vi "roboLV.vi"() -> ()   [LabVIEW 2013]
uses:
  <vilib>/Instr/_visa.llb/VISA Configure Serial Port (Instr).vi
panel:
  out "Elbow Waveform":dbl(graph)
  out "Elbow":dbl[](array[numeric])
  out "Gripper":bool
  out "Wrist":bool
  out "Elbow":bool
  out "Shoulder":bool
  out "Base":bool
  out "Wrist Waveform":dbl(graph)
  out "Shoulder Waveform":dbl(graph)
  out "String":string
  out "Numeric":dbl
  out "Wrist":dbl[](array[numeric])
  out "Shoulder":dbl[](array[numeric])
  in  "Clear":bool
  in  "?":bool
  out "?":bool
  out "Motor":u32
  in  "VISA resource name":refnum<visa-resource-name>
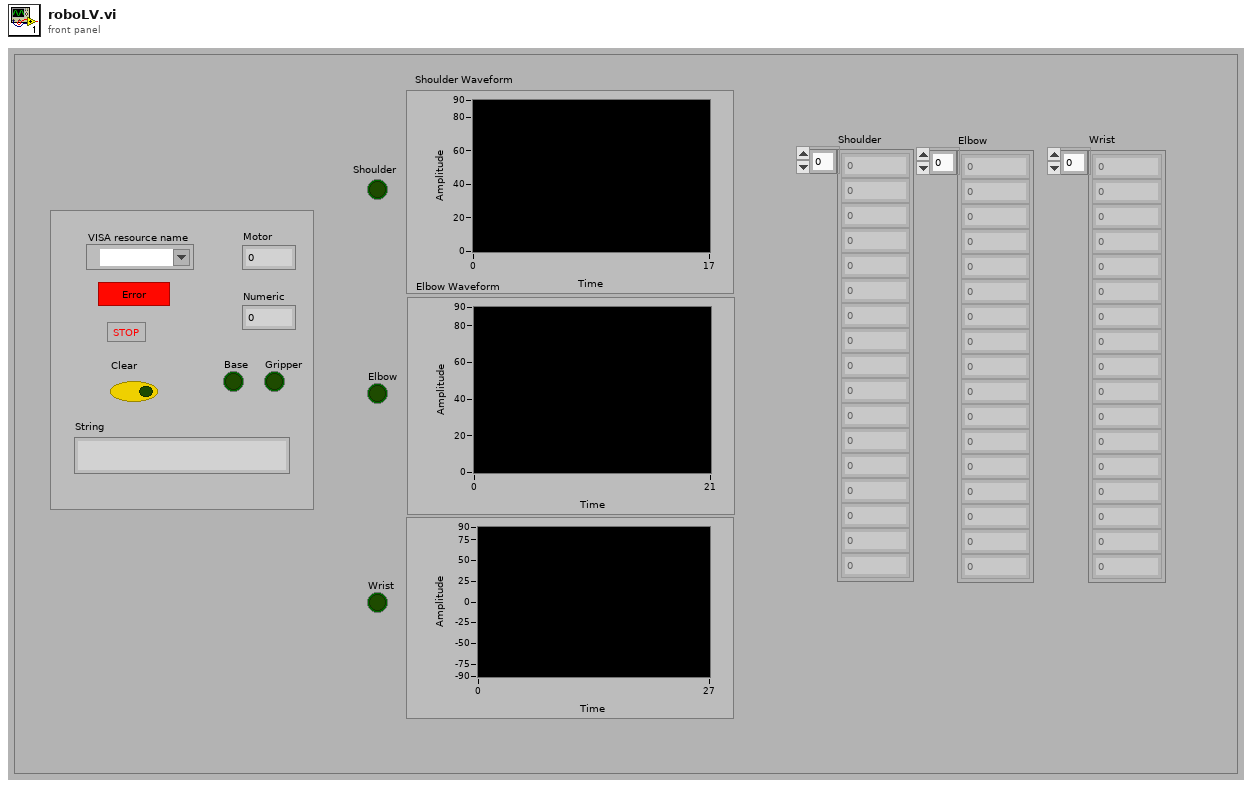
[diagram p1: front panel]
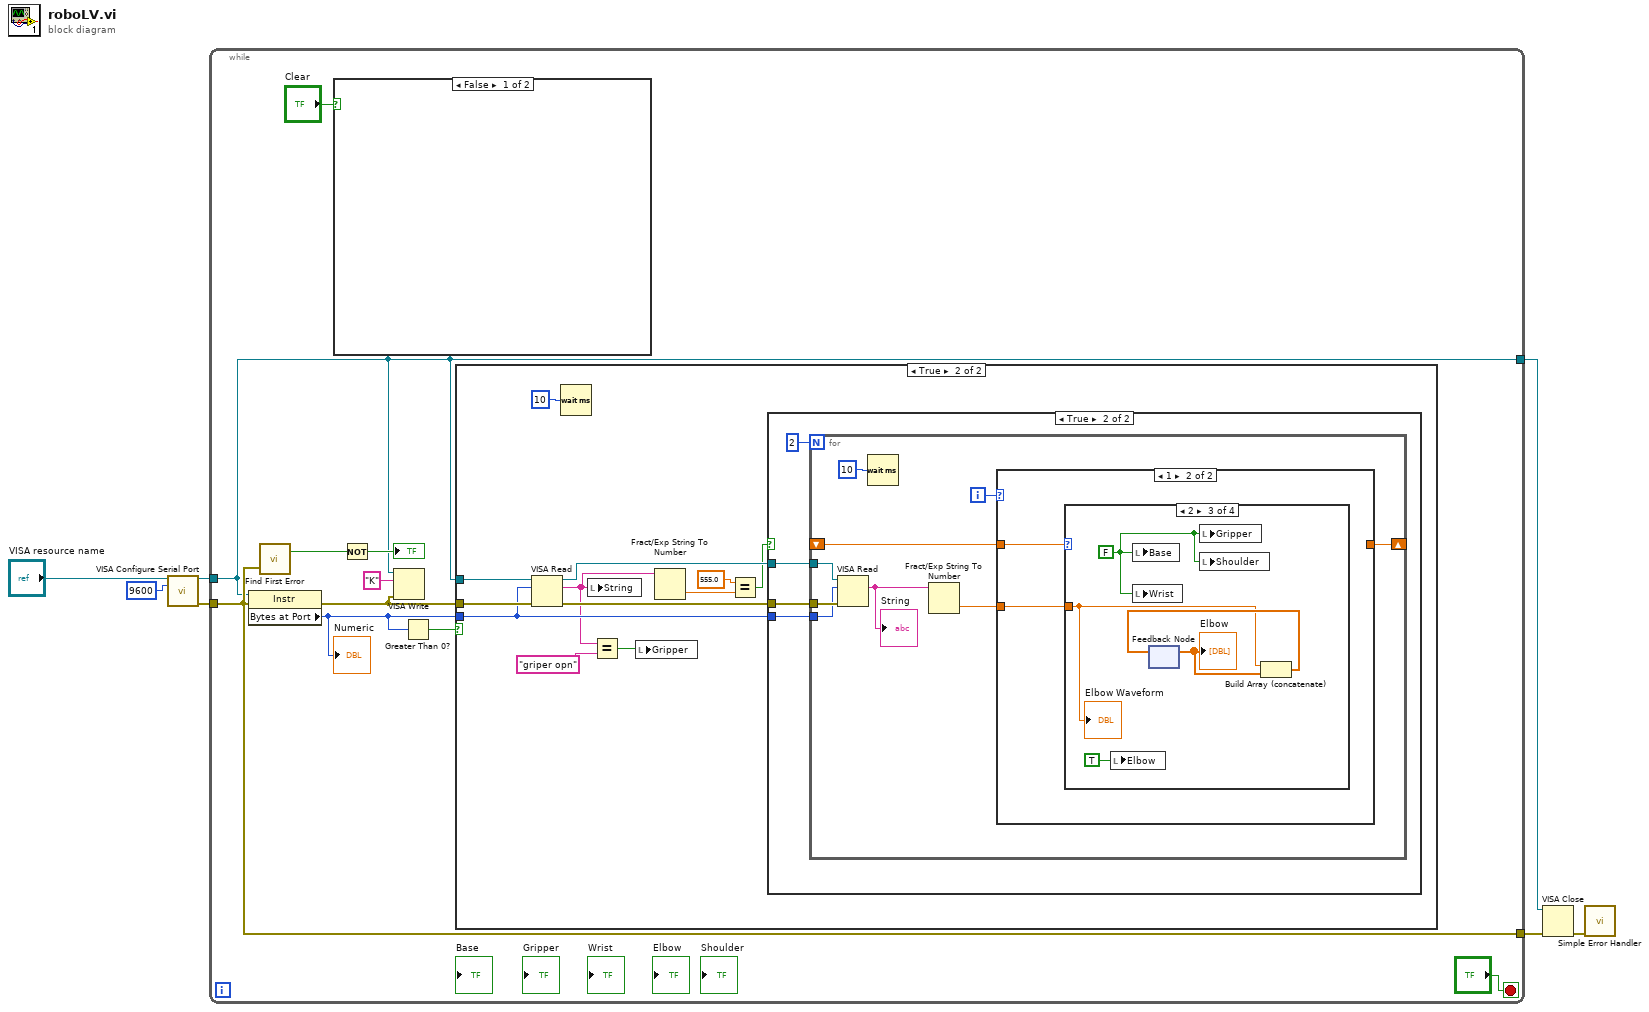
[diagram p0: block diagram]
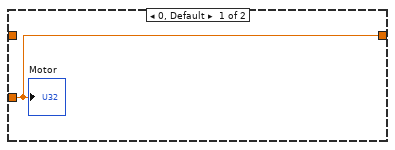
[diagram p4: hidden frame]
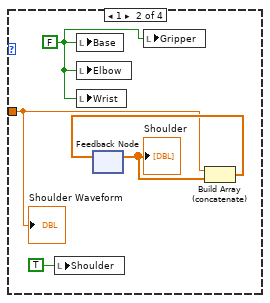
[diagram p6: hidden frame]
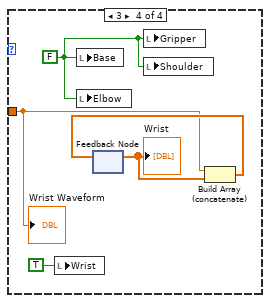
[diagram p7: hidden frame]
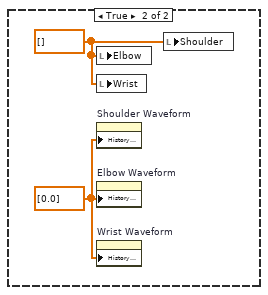
[diagram p8: hidden frame]
diagram:
  n1 = call-poly "VISA Configure Serial Port"("VISA resource name"="VISA resource name", "baud rate (9600)"=u32 9600) -> ("VISA resource name out"=w3:refnum<visa-resource-name>, "error out"=w4:errorcluster)  [unwired: 12 in]
  n2 = while {
    tunnel: w4 -> [w15]
    tunnel: w3 -> [w12]
    tunnel: [w15] -> w2
    tunnel: [w12] -> w1
    stop <- "?" stop-if-true
    n3 = property class="Instr"(reference=w12, error in=w15) -> (error out=w11:errorcluster, "Bytes at Port"=w8:u32)  [unwired: 1 out]
    "Numeric" <- w8
    n4 = call <vilib>:"Find First Error.vi"("error in (no error)"=w15) -> ("error?"=w17:bool)  [unwired: 3 in, 1 out]
    n5 = case shown="False" "Clear" {
      frame False {
      }
      frame True {
        w62 = dbl[] [0.0] ("History Data")
        w61 = dbl[] [] ("History Data")
        n6 = local write "Elbow"(w61) -> ()
        n7 = local write "Wrist"(w61) -> ()
        n8 = property on="Shoulder Waveform" class="WFChart (strict)"("History Data"=w62) -> ()  [unwired: 2 in, 2 out]
        n9 = property on="Elbow Waveform" class="WFChart (strict)"("History Data"=w62) -> ()  [unwired: 2 in, 2 out]
        n10 = property on="Wrist Waveform" class="WFChart (strict)"("History Data"=w62) -> ()  [unwired: 2 in, 2 out]
        n11 = local write "Shoulder"(w61) -> ()
      }
    }
    n12 = Not(x=w17) -> (.not. x?=→"?":bool)
    n13 = VISA Write(VISA resource name=w12, write buffer="K", error in (no error)=w11) -> ()  [unwired: 3 out]
    n14 = Greater Than 0?(x=w8) -> (x > 0?=w10:bool)
    n15 = case shown="True" w10 {
      tunnel: w8 -> [_ w25]
      tunnel: w12 -> [_ w26]
      tunnel: w11 -> [_ w28]
      frame False {
      }
      frame True {
        n16 = VISA Read(VISA resource name=w26, byte count=w25, error in (no error)=w28) -> (VISA resource name out=w27:refnum<visa-resource-name>, read buffer=w20:string, error out=w29:errorcluster)  [unwired: 1 out]
        n17 = Wait (ms)(milliseconds to wait=u32 10) -> ()  [unwired: 1 out]
        n18 = local write "String"(w20) -> ()
        n19 = Equal?(x=w20, y="griper opn") -> (x = y?=w18:bool)
        n20 = local write "Gripper"(w18) -> ()
        n21 = Fract/Exp String To Number(string=w20) -> (number=w23:dbl)  [unwired: 3 in, 1 out]
        n22 = Equal?(x=555.0, y=w23) -> (x = y?=w24:bool)
        n23 = case shown="True" w24 {
          tunnel: w29 -> [_ w32]
          tunnel: w27 -> [_ w31]
          tunnel: w25 -> [_ w30]
          frame False {
          }
          frame True {
            n24 = for {
              N: 2 -> [_]
              tunnel: w31 -> [w42]
              tunnel: w32 -> [w41]
              tunnel: w30 -> [w40]
              shift-right: [w36] -> _
              shift-left: _ -> [w35]
              i -> [w39]
              n25 = VISA Read(VISA resource name=w42, byte count=w40, error in (no error)=w41) -> (read buffer=w37:string)  [unwired: 3 out]
              "String" <- w37
              n26 = Wait (ms)(milliseconds to wait=u32 10) -> ()  [unwired: 1 out]
              n27 = Fract/Exp String To Number(string=w37) -> (number=w38:dbl)  [unwired: 3 in, 1 out]
              n28 = case shown="1" w39 {
                tunnel: w38 -> [w43 w44]
                tunnel: [w43 _] -> w36
                tunnel: w35 -> [_ w45]
                frame 0, Default {
                  "Motor" <- w43
                }
                frame 1 {
                  n29 = case shown="2" w45 {
                    tunnel: w44 -> [_ w49 w54 w58]
                    frame 0, Default {
                    }
                    frame 1 {
                      w47 = FALSE ("Base")
                      n30 = local write "Shoulder"(TRUE ("Shoulder")) -> ()
                      n31 = local write "Base"(w47) -> ()
                      n32 = local write "Elbow"(w47) -> ()
                      n33 = local write "Wrist"(w47) -> ()
                      n34 = feedback #1() -> (w46:dbl[])  [unwired: 1 in]
                      "Shoulder" <- w46
                      n35 = local write "Gripper"(w47) -> ()
                      n36 = Build Array (concatenate)(w49, w46) -> (w50:dbl[])
                      n37 = feedback-in #1(w50) -> ()
                      "Shoulder Waveform" <- w49
                    }
                    frame 2 {
                      w52 = FALSE ("Base")
                      n38 = local write "Elbow"(TRUE ("Shoulder")) -> ()
                      n39 = local write "Base"(w52) -> ()
                      n40 = local write "Wrist"(w52) -> ()
                      n41 = feedback #2() -> (w51:dbl[])  [unwired: 1 in]
                      "Elbow" <- w51
                      n42 = local write "Gripper"(w52) -> ()
                      n43 = local write "Shoulder"(w52) -> ()
                      n44 = Build Array (concatenate)(w54, w51) -> (w55:dbl[])
                      n45 = feedback-in #2(w55) -> ()
                      "Elbow Waveform" <- w54
                    }
                    frame 3 {
                      w56 = FALSE ("Base")
                      n46 = local write "Wrist"(TRUE ("Shoulder")) -> ()
                      n47 = local write "Base"(w56) -> ()
                      n48 = local write "Elbow"(w56) -> ()
                      n49 = feedback #3() -> (w59:dbl[])  [unwired: 1 in]
                      "Wrist" <- w59
                      n50 = local write "Gripper"(w56) -> ()
                      n51 = local write "Shoulder"(w56) -> ()
                      n52 = Build Array (concatenate)(w58, w59) -> (w60:dbl[])
                      n53 = feedback-in #3(w60) -> ()
                      "Wrist Waveform" <- w58
                    }
                  }
                }
              }
            }
          }
        }
      }
    }
  }
  n54 = VISA Close(VISA resource name=w1, error in (no error)=w2) -> (error out=w5:errorcluster)
  n55 = call <vilib>:"Simple Error Handler.vi"("error in (no error)"=w5) -> ()  [unwired: 4 in, 5 out]
